vi "Refname to String (Swerve).vi"(5 "Enum":T1) -> (2 "String":string)   [LabVIEW 2016]
uses:
  Swerve Motors.ctl
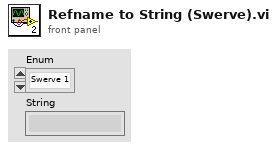
[diagram p1: front panel]
types:
  T1 = typedef "Swerve Motors.ctl" = enum16{"Swerve 1", "Swerve 2", "Swerve 3", "Swerve 4"}
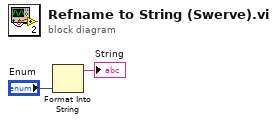
[diagram p0: block diagram]
diagram:
  n1 = Format Into String("Enum") -> (resulting string=→"String":string)  [unwired: 3 in, 1 out]
